vi "配置控件.vi"(8 "error in (no error)":errorcluster caption="错误输入（无错误）", 10 "鼠标位置":T1 caption="点32", 11 "程序响应 输入":refnum<class "程序响应.lvclass">) -> (0 "error out":errorcluster caption="错误输出", 3 "程序响应 输出":refnum<class "程序响应.lvclass">)   [LabVIEW 2018, in "程序响应.lvlib" / "程序响应.lvclass"]
uses:
  <vilib>/Utility/miscctls.llb/LVPoint32TypeDef.ctl
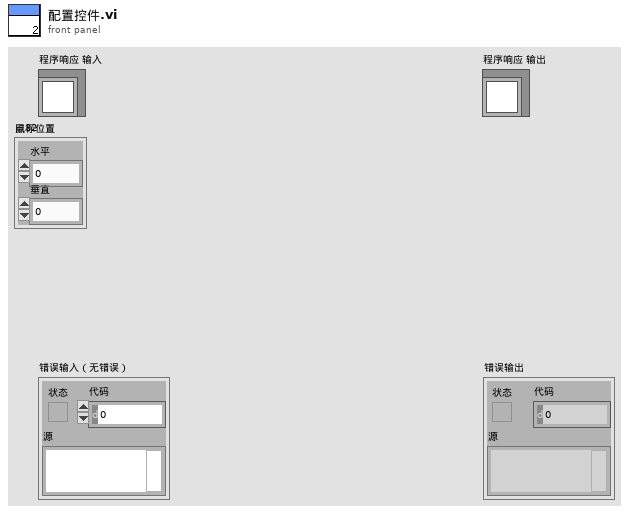
[diagram p1: front panel]
types:
  T1 = typedef "LVPoint32TypeDef.ctl" = cluster{"Horizontal":i32, "Vertical":i32}
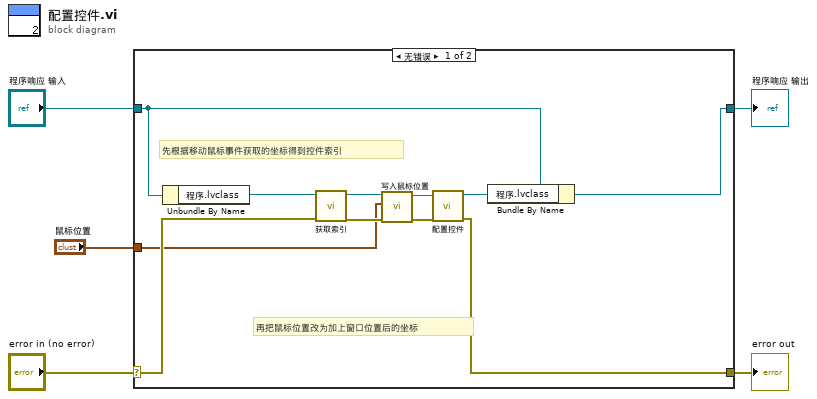
[diagram p0: block diagram]
diagram:
  n1 = case shown="无错误" "error in (no error)" {
    selector: "error in (no error)" -> [w7 w18]
    tunnel: [w13 w18] -> w4
    tunnel: [w14 w17] -> w2
    tunnel: "程序响应 输入" -> [w16 w17]
    tunnel: "鼠标位置" -> [w6 _]
    frame No Error {
      # "再把鼠标位置改为加上窗口位置后的坐标"
      # "先根据移动鼠标事件获取的坐标得到控件索引"
      n2 = Unbundle By Name(w16) -> ("程序.lvclass"=w12:refnum<class "程序.lvclass">)
      n3 = call-dynamic "获取索引.vi"("error in (no error)"=w7, "程序 输入"=w12) -> ("error out"=w8:errorcluster, "程序 输出"=w11:refnum<class "程序.lvclass">)  [unwired: 8 in]
      n4 = call-dynamic "写入鼠标位置.vi"("error in (no error)"=w8, "Point32"=w6, "程序输入"=w11) -> ("error out"=w9:errorcluster, "程序输出"=w10:refnum<class "程序.lvclass">)  [unwired: 7 in]
      n5 = call-dynamic "配置控件.vi"("error in (no error)"=w9, "程序 输入"=w10) -> ("error out"=w13:errorcluster, "程序 输出"=w15:refnum<class "程序.lvclass">)  [unwired: 8 in]
      n6 = Bundle By Name(cluster=w16, "程序.lvclass"=w15) -> (w14:refnum<class "程序响应.lvclass">)
    }
    frame Error {
    }
  }
  "error out" <- w4
  "程序响应 输出" <- w2
